vi "2024_day06_Task02.vi"() -> ()   [LabVIEW 2023]
uses:
  <userlib>/_OpenG.lib/array/array.llb/Search 1D Array (Variant)__ogtk.vi
  <userlib>/_OpenG.lib/string/string.llb/openg_string.lvlib
  <userlib>/_OpenG.lib/array/array.llb/openg_array.lvlib
panel:
  out "Numeric 2":i32
  out "Numeric":i32
  out "Array":i32[][](array[numeric])
  out "Result - Task 2":i32
  in  "Switch":bool caption="Ex. Data  vs.  User Data"
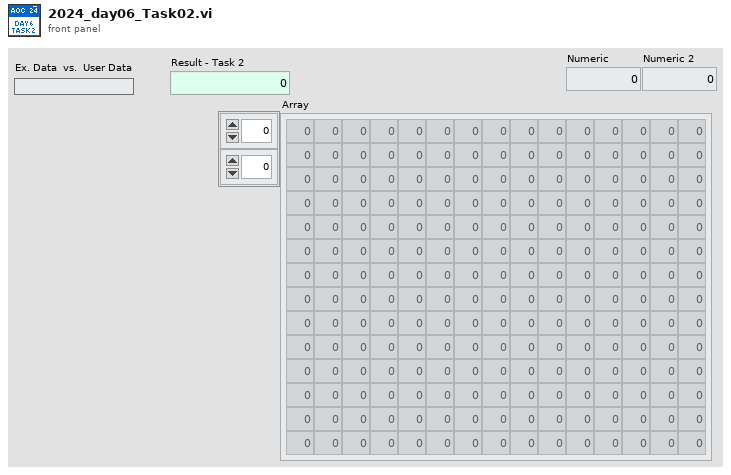
[diagram p1: front panel]
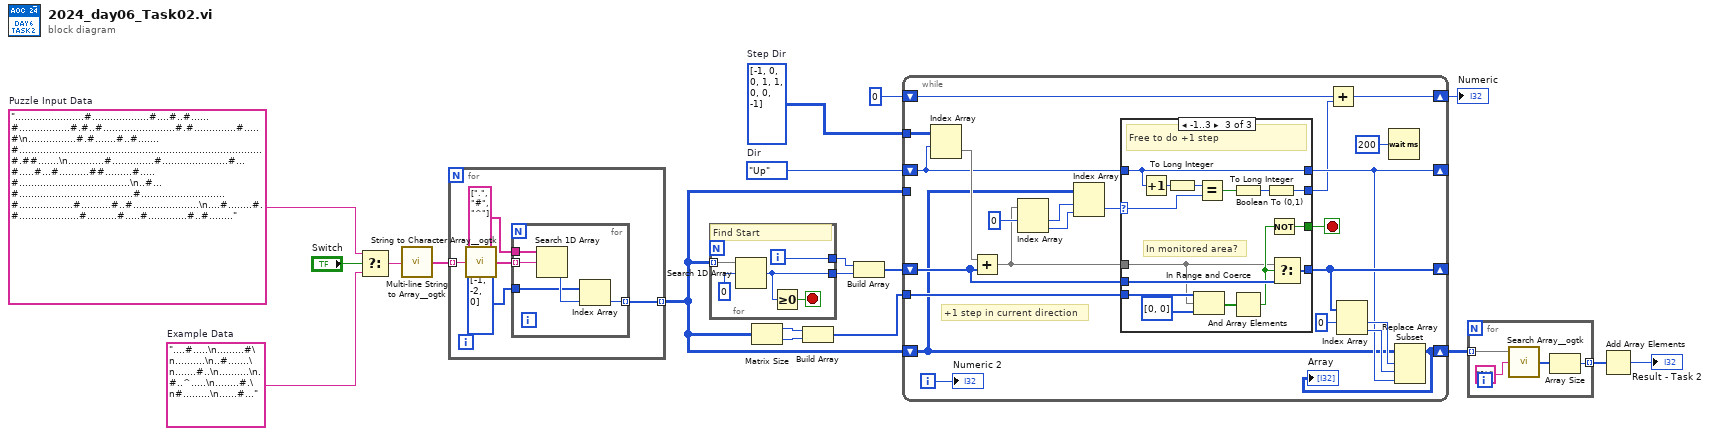
[diagram p0: block diagram]
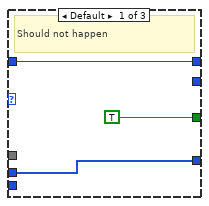
[diagram p2: hidden frame]
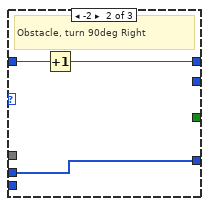
[diagram p3: hidden frame]
diagram:
  w11 = i32[][] [[-1, 0], [0, 1], [1, 0], [0, -1]]  # Step Dir
  w14 = enum16{"Up", "Right", "Down", "Left"}."Up"  # Dir
  w17 = ".......................#...................#....#..#......#.................#.#..#........................#.#..............#.....#\n................#.#.......#..#.......#.................................................................................#.##.......\n............#..............#......................#...#.....#...#..........##.........#.....#.....................................\n..#...#......................................#............................#..................#..........#..#......................\n....#........#.#....................#..........#.....#.............#..#............................#..................#......#....\n..........................................................#................#............................................#.........\n..#............................#.....#...........................#...........#........##...........................#..#...........\n.....................#...........................#.#..............#......................................#.........#....#.....#...\n.#...#.#.................#....................#...............................................................#.#..........#......\n....#....................................#...........................................#.....#..........#...........................\n.......................#..........#..............#......#....#.......#........................................#.#.................\n......#...........................................................#...#............#.................#............................\n.......#.................#..#.....................#...............................................................................\n..............#....................#.#..........#........#......#................#.................#..........#...................\n#.#.......................................#.........................#...................................#.........................\n...#.........................................................................................#................#..................#\n#.....#....#............................................................#.........................#..................#.#..........\n.#.....#.#.......#.#..................#.#......................#.......#.....#..#..................##.....#.......#...#...........\n....#.........#.................................#..........#........#...............#................#...................#....#...\n.................#...............#...#.................#.................................................#........................\n....#...#...............................#..................................................#..........#................#.....#....\n...........#........#....#.......#...#..........#...............#.....#.....#.....#..........#....................................\n............#.........#.................#................#.................#.#..................................................#.\n............#......................................#...................................................................#..........\n...........#....#.....................................................................................#............#..........#...\n..........#........................................#.............#.................#........................#..#.......#........#.\n......#.............................#.................##..................................#.....................#.................\n.#.................................#.............................................#.................##.....#..............#......#.\n.........................#..............................#..........#...........#....#................#......................#.....\n.......#...................#......##........................#.........#...........................................................\n......................................................................##...........#................#.............................\n....#...................................##...............................................#........................................\n...##.....#..#........#.................#..............................................................#..........................\n........##......#....................#..............................#......................#...................#..................\n.........................................................#.......................................................#.#..............\n..........#.............................#.........#...............#................#.#.........#..........................#.#.....\n....................#...................#..#.......................................................#..........#...............#...\n...........................................................#........................#.........#........#..........................\n.......#..............#......#.................................#...................##...........................#.........#.......\n#...#...............................................................................................................#.............\n................................#..#....#............#...........#..................#.............................#...............\n....................#..............#.........#.................................#.............#..##................................\n#...#..................................................................................#.....#...........#........................\n........#...........#........#...#..................#.....#....#.........#.........................#...........................#..\n.............#...#...................................................................#...........#................................\n.............#........................................#...#.............#..............................#..#.........#.............\n...#.................................................................................#.............#..........................##..\n...#..............................................................................................................................\n................#.........#..................................#...................#................................................\n...#................#...#.#.....................#...........#..................................#........#....#......#.............\n..........................#.....................#..#...................................##........................................#\n#........................#...............................................#........#..#..........#...........................#.....\n.#............#.#..............................................................#...........#......................................\n......#..................................................................#.......#..............................#...#....#........\n........#........................#.........#.............#.....#..................................................................\n...............................................................................#...........................................#......\n........................#..................................#.....................................................#................\n............................................................#..........................#.................#.......................#\n.....................#..#.........................#..............#.............................#........#..............##......#..\n.....................#.................................................#.......#............#........................#.......#....\n......................#.....................................................#......#............................#.................\n................................................................#...#..##..#.....................................#...............#\n..............#..............................................................................................#....................\n............................................#......#..........#...............................................................#...\n....#.................................#..................................................................#..........##..#.........\n............#.....#................................................................................#..........#.........#.........\n.....................#......................................#.........#....................................................#....#.\n.........................#...............................#...............................#....................#...................\n.#.....................#.#.......................................#....#...........#.......................#.......................\n.....................................................#.#..#......................................................................#\n#..........#..........................#............................#.............#..................#.............#...........#...\n........#.........................................................................................................................\n..........#.............#.........................................#................................................#..............\n...........#................................#.................#...........................#.............................#.........\n..................#.........................................#.#..................#...#...........#.......#..#.....................\n........................................................#...#.......................................................#.............\n.........................................................................#.......#..#.....#.......................................\n............#..............................................................#.........#..............#.............#...............\n#...#..........................................#...........#.....#.....................................#...............#..........\n...........................#............#.........................................................................................\n...#..........................................#.......................................................................#...........\n..............#......#.....#.....................#..........................#.....................................................\n.........................#....#...................#...#.......#..............................#........................#...........\n.............................#............^.#................................................#......#..#.#...........#............\n....................................................................................#...#.#...................................#...\n.......................#..............................##..............................................#...........................\n......................#...................................................#..........................................#............\n......#........................................................................#.....................................#............\n.......................#.............................#........................#...........#...........#............#...........#..\n....#...............#..#......#....#..................#.............#.......#...............#.......................#.............\n............#...#..................#..............................................................................................\n....#.......#.................#.......................................................#..#......#.................................\n.........#......#..........#......................#.....................#..................#.#....................................\n...............##.......................................................#...#.............................#.......#...............\n........................................................##...................#...#............#......#............................\n...........#...#..............#.............................................................#...................#............#....\n...............................................#.....#.....#......................................................................\n.#....................#...#........#....................#.#.........#..........#................................#................#\n.............#.....#..#....................................#.#...........#.................................................#..#.#.\n......#.....................................#....................................................................#................\n............................................................##......#.....................#.......#.....................#...#.....\n.#.......#......................#.................................................................................................\n................#....#......................#.........#...................#........#.......##.....#...............................\n..#....#....................#............................................................#.#......#............#.....#.#....#.....\n.................................#.................................................#.......#......................................\n..................#...........#....#.....................#......#...............#..................#....................##........\n.##...............................................#............#...........................#......................................\n.............#...........#...........................#..#.......#...#..........#......................#..........#................\n.......#...................................#.................#....#..............................................................#\n........#....................................................#.................#.....#.........#.#................................\n................#.................................#.....................#.....#.....#............................##...............\n..............................................##.................#..##........#...........#............#..........................\n....#......................................#...............................................................................#......\n..#..............#.#................#..#..............#.......................................#.#.......#..............#......#..#\n.....#..............................................................................................................#.......#.....\n..#.......#.#..........#.......#..................................#..........#.......#.................#...........#...........#..\n...............#.....#................#............#................#............#.....#.#........#...............................\n....#.....................#................#.....................................#......................#.#.......#....#..........\n........#...............#...#.....................................................#........#.........#.........#..................\n...#......#..........................#.....#..........................##.......#....#.............................................\n.............#................................#............................#.....#.......#......#................................#\n.......................#............#..........................#..................................................................\n.................................................#..............#...#...........................#.................................\n......#...................#..............................................................................................#....#..#\n....................................#......#.....................#..............#.......#...................#.....................\n............#...................................#...........#........#........#...........................................##......\n#...........#..........................#....................................#.........#................................#..........\n......##..#...............................................................#...............................#.........#.............\n.......................#.....#.........................#...#.........................#.....#..........#.#...#.....................\n.......................#..#.....#.....#..........................#.........#.....#....................#.....#....................#"  # Puzzle Input Data
  w18 = "....#.....\n.........#\n..........\n..#.......\n.......#..\n..........\n.#..^.....\n........#.\n#.........\n......#..."  # Example Data
  n1 = Select(t=w17, s="Switch", f=w18) -> (s? t:f=w16:string)
  n2 = call <userlib>:"Multi-line String to Array__ogtk.vi"("string"=w16) -> ("lines"=w15:string[])
  n3 = for {
    tunnel: w15 -> [w24] mode=indexing
    tunnel: [w20] -> w3 mode=indexing
    n4 = call <userlib>:"String to Character Array__ogtk.vi"("Input String"=w24) -> ("Character Array"=w23:string[])
    n5 = for {
      tunnel: w23 -> [w29] mode=indexing
      tunnel: string[] [".", "#", "^"] -> [w28]
      tunnel: i32[] [-1, -2, 0] -> [w26]
      tunnel: [w25] -> w20 mode=indexing
      n6 = Search 1D Array(1D array=w28, element=w29) -> (index of element=w27:i32)  [unwired: 1 in]
      n7 = Index Array(array=w26, index=w27) -> (element=w25:i32)
    }
  }
  n8 = for {
    tunnel: [w33] -> w13
    tunnel: [w32] -> w12
    tunnel: w3 -> [w31] mode=indexing
    i -> [w32]
    stop <- w34 stop-if-true
    # "Find Start"
    n9 = Search 1D Array(1D array=w31, element=0) -> (index of element=w33:i32)  [unwired: 1 in]
    n10 = Greater Or Equal To 0?(x=w33) -> (x >= 0?=w34:bool)
  }
  n11 = Matrix Size(0:w3) -> (1:w6:i32, 2:w5:i32)
  n12 = Build Array(w6, w5) -> (w4:i32[])
  n13 = Build Array(w12, w13) -> (w8:i32[])
  n14 = while {
    tunnel: w3 -> [_]
    shift-right: [w44] -> _
    shift-left: w8 -> [w50]
    shift-right: [w43] -> _
    shift-left: w14 -> [w51]
    tunnel: w11 -> [w57]
    shift-right: [w40] -> w9
    shift-left: w3 -> [w35]
    tunnel: w4 -> [w42]
    shift-right: [w38] -> w1
    shift-left: 0 -> [w39]
    i -> [w36]
    stop <- w48 stop-if-true
    # "+1 step in current direction"
    n15 = Index Array(array=w57, index (row)=w51) -> (element=w56:i32[])  [unwired: 1 in]
    n16 = Add(x=w56, y=w50) -> (x+y=w49:i32[])
    n17 = Index Array(array=w49, index #1=0 ("index")) -> (element #1=w54:i32, element #2=w53:i32)  [unwired: 1 in]
    n18 = Index Array(array=w35, index (row)=w54, index (col)=w53) -> (element=w52:i32)
    n19 = case shown="-1..3" w52 {
      selector: w52 -> [_ _ w68]
      tunnel: [w60 w62 w70] -> w43
      tunnel: w51 -> [w60 w63 w70]
      tunnel: [w59 w61 w77] -> w44
      tunnel: w50 -> [w59 w61 w78]
      tunnel: w49 -> [_ _ w71]
      tunnel: [TRUE _ w73] -> w48
      tunnel: w42 -> [_ _ w76]
      tunnel: [_ _ w64] -> w37
      frame Default {
        # "Should not happen"
      }
      frame -2 {
        # "Obstacle, turn 90deg Right"
        n20 = Increment(x=w63) -> (x+1=w62:enum16{"Up", "Right", "Down", "Left"})
      }
      frame -1..3 {
        # "In monitored area?"
        # "Free to do +1 step"
        n21 = Increment(x=w70) -> (x+1=w69:enum16{"Up", "Right", "Down", "Left"})
        n22 = To Long Integer(number=w69) -> (32bit integer=w67:i32)
        n23 = In Range and Coerce(upper limit=w76, x=w71, lower limit=i32[] [0, 0]) -> (In Range?=w75:bool[])  [unwired: 1 out]
        n24 = Equal?(x=w67, y=w68) -> (x = y?=w66:bool)
        n25 = Boolean To (0,1)(Boolean=w66) -> (0, 1=w65:i16)
        n26 = And Array Elements(Boolean array=w75) -> (logical AND=w72:bool)
        n27 = To Long Integer(number=w65) -> (32bit integer=w64:i32)
        n28 = Not(x=w72) -> (.not. x?=w73:bool)
        n29 = Select(t=w71, s=w72, f=w78) -> (s? t:f=w77:i32[])
      }
    }
    n30 = Add(x=w39, y=w37) -> (x+y=w38:i32)
    n31 = Index Array(array=w44, index #1=0 ("index")) -> (element #1=w46:i32, element #2=w45:i32)  [unwired: 1 in]
    n32 = Wait (ms)(milliseconds to wait=u32 200) -> ()  [unwired: 1 out]
    n33 = Replace Array Subset(array=w35, new element=w43, index (row)=w46, index (col)=w45) -> (w40:i32[][])
    "Array" <- w40
    "Numeric 2" <- w36
  }
  "Numeric" <- w1
  n34 = for {
    tunnel: w9 -> [w82] mode=indexing
    tunnel: [w79] -> w10 mode=indexing
    n35 = call-poly <userlib>:"Search Array__ogtk.vi"("Array"=w82, "Element Data"="%" ("new element/subarray")) -> ("Indices of Elements"=w80:i32[])  [unwired: 7 in]
    n36 = Array Size(array=w80) -> (size(s)=w79:i32)
  }
  n37 = Add Array Elements(numeric array=w10) -> (sum=→"Result - Task 2":i32)
